vi "Ctor.vi"(8 "error in (no error)":errorcluster) -> (0 "error out":errorcluster, 3 "Tread out":refnum<class "Tread.lvclass">)   [LabVIEW 2020, in "Tread.lvclass"]
uses:
  Tread.lvclass
  Ref Data.ctl
  Location.ctl
  bno055/BNO055/BNO055/Address.ctl
  bno055/BNO055/BNO055/Operating Mode.ctl
  Tread.lvclass/Tread.ctl
  <vilib>/MakerHub/LINX/Public/Utilities/Open Local.vi
  <vilib>/MakerHub/LINX/LMH-LINX.lvlib
  nmea/nmea/VISA GPS/VISA GPS.lvclass
  bno055/BNO055/BNO055/BNO055.lvclass
  lv-parallax-lcd/Parallax LCD/LCD/LCD.lvclass
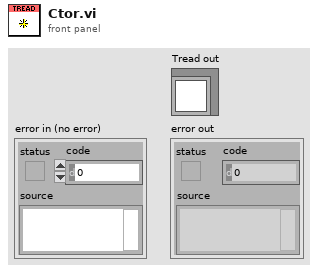
[diagram p1: front panel]
types:
  T1 = typedef "BNO055.lvlib/BNO055.lvclass/Operating Mode.ctl" = enum8{"Config", "Acc Only", "Mag Only", "Gyr Only", "Acc Mag", "Acc Gyr", "Mag Gyr", "AccMagGyr", "IMU", "Compass", "Mag4Gyr", "NDOF FMC Off", "NDOF"}
  T2 = typedef "BNO055.lvlib/BNO055.lvclass/Address.ctl" = u8
  T3 = typedef "Tread.lvclass/Ref Data.ctl" = cluster{"Current Loc":T4, "Goal Loc":T4, "Current Heading":dbl, "Goal Heading":dbl, "Goal Distance":dbl, "Goal Threshold":dbl}
  T4 = typedef "Tread.lvclass/Location.ctl" = cluster{"Lat":dbl, "Lon":dbl}
  T5 = typedef "LMH-LINX.lvlib/LINX Ref.ctl" = cluster{"IO":T6, "Interface":T7, "LINX Device Config":T8}
  T6 = typedef "LMH-LINX.lvlib/Platform.ctl" = enum16{"Remote", "Local"}
  T7 = typedef "LMH-LINX.lvlib/Interface.ctl" = enum16{"Serial", "TCP"}
  T8 = typedef "LMH-LINX.lvlib/Device.lvlib/LINX Device Config.ctl" = cluster{"Interface":T7, "COM Port":refnum<visa-resource-name>, "TCP Configuration":T9, "Device Family":u8, "Device ID":u8, "Device Name":string, "TCP Ref":refnum<k5>, "Channels":T10}
  T9 = typedef "LMH-LINX.lvlib/Device.lvlib/TCP Config.ctl" = cluster{"IP Address":string, "Port":u16}
  T10 = typedef "LMH-LINX.lvlib/Channels.ctl" = cluster{"DI":u8[], "DO":u8[], "AI":u8[], "AO":u8[], "PWM":u8[], "QE":u8[], "UART":u8[], "I2C 2":u8[], "SPI":u8[], "CAN":u8[], "Servo":u8[], "AI Ref (V)":dbl, "AI Resolution (Bits)":u8, "AO Ref (V)":dbl, "AO Resolution (Bits)":u8}
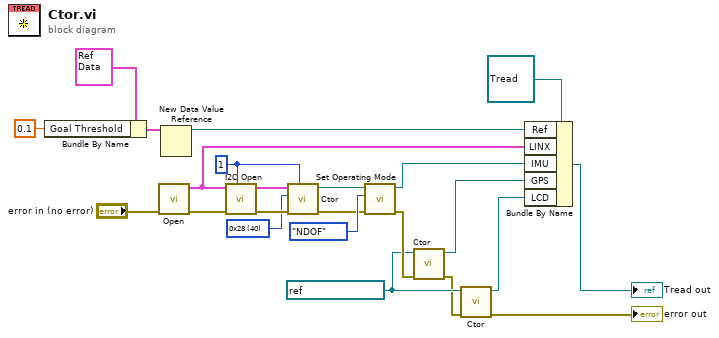
[diagram p0: block diagram]
diagram:
  w13 = T2 40 items=["0x28"=40, "0x29"=41] ("Address")
  w14 = u8 1 ("I2C Channel (0)")
  w4 = refnum<visa-resource-name> "ASRL1::INSTR" ("VISA Port")
  n1 = Bundle By Name(cluster=T3 {"Current Loc"={"Lat"=0.0, "Lon"=0.0}, "Goal Loc"={"Lat"=0.0, "Lon"=0.0}, "Current Heading"=0.0, "Goal Heading"=0.0, "Goal Distance"=0.0, "Goal Threshold"=0.0} ("Ref Data"), "Goal Threshold"=0.1) -> (w11:T3)
  n2 = call-poly <vilib>:"Open.vi"("Error In"="error in (no error)") -> ("Error Out"=w17:errorcluster, "LINX Resource"=w18:T5)  [unwired: 8 in, 1 out]
  n3 = New Data Value Reference(data value=w11) -> (data value reference=w20:refnum<data-value>)  [unwired: 1 in, 1 out]
  n4 = call <vilib>:"I2C Open.vi"("I2C Channel (0)"=w14, "Error In"=w17, "LINX Resource"=w18) -> ("Error Out"=w16:errorcluster, "LINX Resource"=w15:T5)  [unwired: 7 in]
  n5 = call "Ctor.vi"("I2C Channel"=w14, "error in (no error)"=w16, "Address"=w13, "LINX Resource"=w15) -> ("error out"=w7:errorcluster, "BNO055 out"=w9:refnum<class "BNO055.lvclass">)  [unwired: 5 in, 1 out]
  n6 = call "Set Operating Mode.vi"("error in (no error)"=w7, "Operating Mode"=Operating_Mode."NDOF", "BNO055 in"=w9) -> ("error out"=w5:errorcluster, "BNO055 out"=w6:refnum<class "BNO055.lvclass">)  [unwired: 7 in]
  n7 = call "Ctor.vi"("error in (no error)"=w5, "VISA Port"=w4) -> ("error out"=w3:errorcluster, "VISA GPS out"=w19:refnum<class "VISA GPS.lvclass">)  [unwired: 8 in]
  n8 = call "Ctor.vi"("error in (no error)"=w3, "VISA Port"=w4) -> ("error out"=→"error out":errorcluster, "LCD out"=w2:refnum<class "LCD.lvclass">)  [unwired: 8 in]
  n9 = Bundle By Name(cluster=refnum<class "Tread.lvclass"> refnum ("Tread in"), "Ref"=w20, "LINX"=w18, "IMU"=w6, "GPS"=w19, "LCD"=w2) -> (→"Tread out":refnum<class "Tread.lvclass">)
